vi "Remove Subordinate.vi"(8 "error in (no error)":errorcluster, 10 "Identifier":string, 11 "Managed Actor in":refnum<class "Managed Actor.lvclass">) -> (0 "error out":errorcluster, 3 "Managed Actor out":refnum<class "Managed Actor.lvclass">)   [LabVIEW 2023, in "Engine.lvlib" / "Managed Actor.lvlib" / "Managed Actor.lvclass"]
doc: "<b>Remove Subordinate</b> is to dynamically shut down actors. The routine deletes the actor from the map and transmits a stop command to the subordinate actor. IF the actor is not found, a warning is thrown indicating the actor was not found."
uses:
  Library/Managed Actor.lvclass
  Library/Managed Actor.lvclass/Managed Actor.ctl
  <vilib>/Utility/error.llb/Error Cluster From Error Code.vi
  <vilib>/ErrorRing/Error Ring.xnode
  builds/Framework/Actor Framework.lvlibp/1abvi3w/vi.lib/ActorFramework/Stop Msg/Stop Msg.lvclass
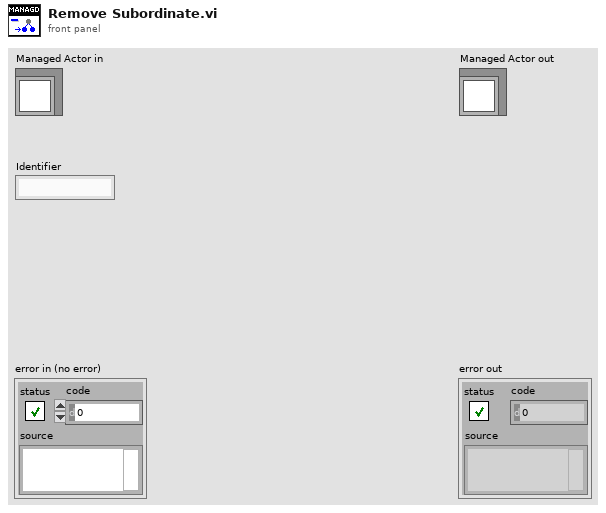
[diagram p1: front panel]
types:
  T1 = typedef "Engine.lvlib/Managed Actor.lvlib/Managed Actor.lvclass/Subordinate.ctl" = cluster{"Identifier":string, "Queue":refnum<class "Message Enqueuer.lvclass">, "PanelIndex":i32}
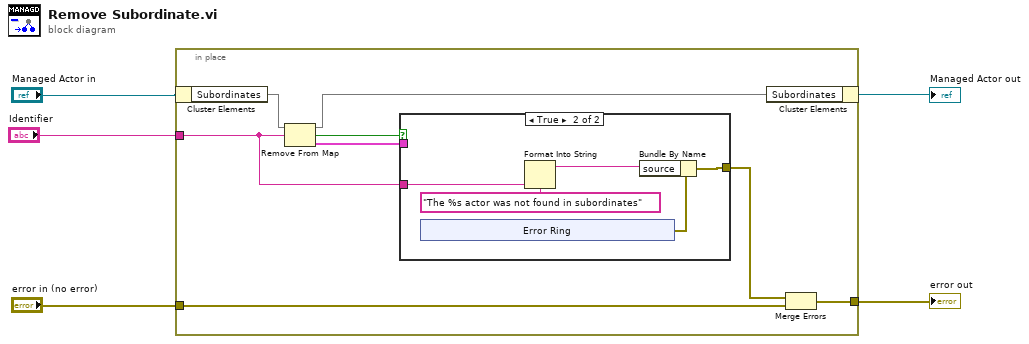
[diagram p0: block diagram]
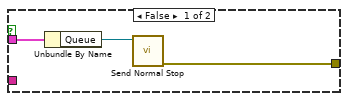
[diagram p2: hidden frame]
diagram:
  n1 = in-place {
    in-place-border: "Identifier" -> [w9]
    in-place-border: "error in (no error)" -> [w6]
    in-place-border: [w7] -> w1
    n2 = in-place-cluster #1("Managed Actor in") -> ("Subordinates"=w13:map{string, T1})
    n3 = Remove From Map(10:w9, 11:w13) -> (1:w10:T1, 2:w11:bool, 3:w12:map{string, T1})
    n4 = case shown="True" w11 {
      tunnel: w10 -> [w16 _]
      tunnel: w9 -> [_ w18]
      tunnel: [w14 w17] -> w8
      frame False {
        n5 = Unbundle By Name(w16) -> ("Queue"=w15:refnum<class "Message Enqueuer.lvclass">)
        n6 = call "Send Normal Stop.vi"("Message Enqueuer"=w15) -> ("error out"=w14:errorcluster)  [unwired: 10 in]
      }
      frame True {
        n7 = xnode "Error Ring"() -> ("error out"=w20:errorcluster)
        n8 = Format Into String(format string="The %s actor was not found in subordinates", w18) -> (resulting string=w21:string)  [unwired: 2 in, 1 out]
        n9 = Bundle By Name(cluster=w20, "source"=w21) -> (w17:errorcluster)
      }
    }
    n10 = in-place-cluster #1("Subordinates"=w12) -> (→"Managed Actor out":refnum<class "Managed Actor.lvclass">)
    n11 = Merge Errors(w8, w6) -> (w7:errorcluster)
  }
  "error out" <- w1
